vi "Set Percentage.vi"(8 "error in (no error)":errorcluster, 10 "Sideways Motors Percentage":dbl(slide) min=-1.0 max=1.0 scale=-1.0..1.0, 11 "Sideways Drive in":refnum<class "Sideways Drive.lvclass">) -> (0 "error out":errorcluster, 3 "Sideways Drive out":refnum<class "Sideways Drive.lvclass">)   [LabVIEW 2014, in "Sideways Drive.lvlib" / "Sideways Drive.lvclass"]
uses:
  Sideways Drive.lvclass
  Sideways Drive.lvclass/Sideways Drive.ctl
  Motor with Encoders/Motors with Encoders Messages/Set Rate (Percent) Msg/Set Rate (Percent) Msg.lvclass/Set Rate (Percent) Msg.ctl
  <vilib>/ActorFramework/Message Enqueuer/Message Enqueuer.lvclass/Message Enqueuer.ctl
  <vilib>/ActorFramework/Message Enqueuer/Enqueue.vi
  <vilib>/ActorFramework/Message Priority Queue/Priority Enqueue.vi
  Motor with Encoders/Motors with Encoders Messages/Set Rate (Percent) Msg/Set Rate (Percent) Msg.lvclass
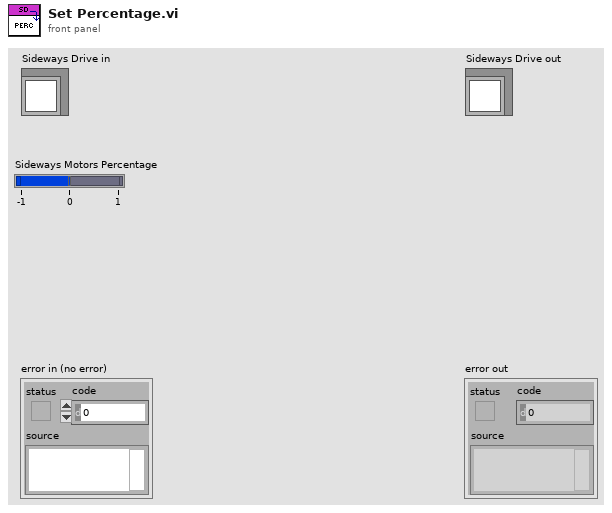
[diagram p1: front panel]
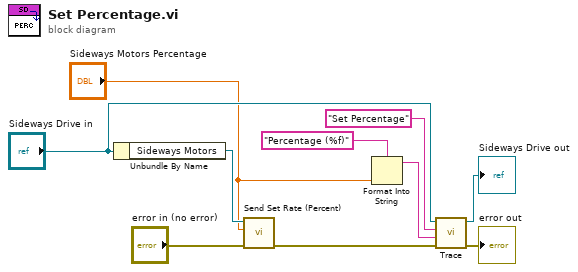
[diagram p0: block diagram]
diagram:
  n1 = Unbundle By Name("Sideways Drive in") -> ("Sideways Motors"=w10:refnum<class "Message Enqueuer.lvclass">)
  n2 = call "Send Set Rate (Percent).vi"("error in (no error)"="error in (no error)", "Rate (Percentage)"="Sideways Motors Percentage", "Message Enqueuer"=w10) -> ("error out"=w5:errorcluster)  [unwired: 7 in, 1 out]
  n3 = Format Into String(format string="Percentage (%f)", "Sideways Motors Percentage") -> (resulting string=w1:string)  [unwired: 2 in, 1 out]
  n4 = call-dynamic "Trace.vi"("error in (no error)"=w5, "System Message"=w1, "System Action"="Set Percentage", "System Actor in"="Sideways Drive in") -> ("error out"=→"error out":errorcluster, "System Actor out"=→"Sideways Drive out":refnum<class "Sideways Drive.lvclass">)  [unwired: 6 in]
